vi "Test Async Handler Warning Logged.vi"(8 "error in (no error)":errorcluster, 11 "Test Case In":refnum<class "Async Handling Test.lvclass">) -> (0 "error out":errorcluster, 3 "Test Case Out":refnum<class "Async Handling Test.lvclass">)   [LabVIEW 2020, in "Async Handling Test.lvclass"]
uses:
  Async Handling Test.lvclass
  C:/Program Files (x86)/National Instruments/LabVIEW 2020/vi.lib/Astemes/LUnit/Test Case.lvclass
  Mock Async Handler Process/Mock Async Handler Process.lvclass
  C:/Git/astemes-triarc-framework/source/Framework/Process/Process.lvclass
  source/Framework Test Suite/Mock Log Handler/Mock Log Handler.lvclass
  C:/Git/astemes-triarc-framework/source/Framework/Logging/Logging.lvclass
  source/Framework/Process/Process.lvclass/Process.ctl
  <vilib>/Astemes/LUnit/Test Case.lvclass/Test Case.ctl
  01074fa8-ee8a-411d-bc8b-fc92c4f90959.vi
  source/Framework/Process/Public/Lifecycle/Get Lifecycle State.vi
  source/Framework/Process/Protected/Messaging/Send Message.vi
  source/Framework/Broadcast Event Helpers/Execution timer.vi
  source/Framework/Process/Private/SubVIs/Wait for finish.vi
  source/Framework/Process/Private/SubVIs/Set Lifecycle State.vi
  <vilib>/Astemes/LUnit/Palette/Pass.vi
  <vilib>/Astemes/LUnit/Palette/Fail.vi
  <vilib>/Astemes/LUnit/Compare Variants.vi
  <vilib>/Astemes/LUnit/Describe Comparison.vi
  <vilib>/Astemes/LUnit/Set Assertion Type.vi
  <vilib>/Utility/error.llb/Clear Errors.vi
  source/Framework/Process/Private/SubVIs/Handle Debug Data.vi
  <vilib>/Astemes/LUnit/Add test result.vi
  <vilib>/Astemes/LUnit/Variant to string.vi
  source/Framework/Logging/Log Debug.vi
  <vilib>/AdvancedString/1D String Array to Delimited String.vi
  <vilib>/Utility/High Resolution Relative Seconds.vi
  <vilib>/Astemes/LUnit/LUnit Record Assertion Result.vi
  <vilib>/Astemes/LUnit/LUnit Aggregate Assertion Results.vi
  <vilib>/Astemes/LUnit/Method Result/LUnit Merge Status.vi
  <vilib>/Astemes/LUnit/LUnit Concatenate result strings.vi
  <vilib>/Utility/error.llb/Error Cluster From Error Code.vi
  source/Framework/Process/Public/Read Name.vi
  source/Framework/Broadcast Event Helpers/Dequeue Broadcast Message.vi
  <vilib>/Utility/Data Type/Get Type Information.vi
  <vilib>/Utility/LVClass/Get LV Class Name.vi
  source/Framework/Process/Process.lvclass
  source/Framework/Broadcast Event Helpers/Broadcast Event Helpers.lvlib
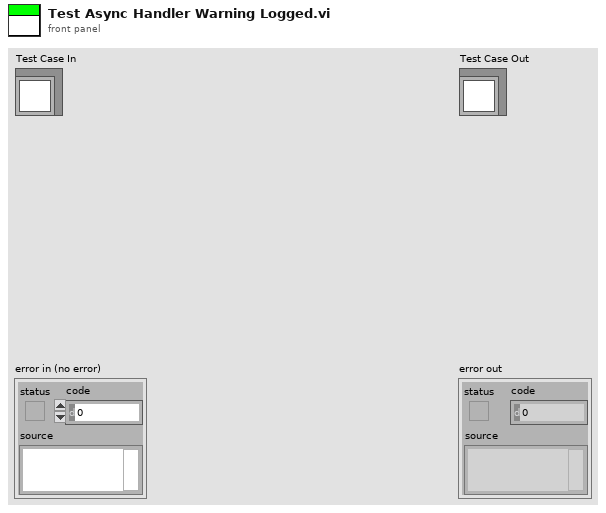
[diagram p1: front panel]
types:
  T1 = typedef "Mock Log Handler.lvclass/Log Entry.ctl" = cluster{"Level":string, "Source":string, "Message":string}
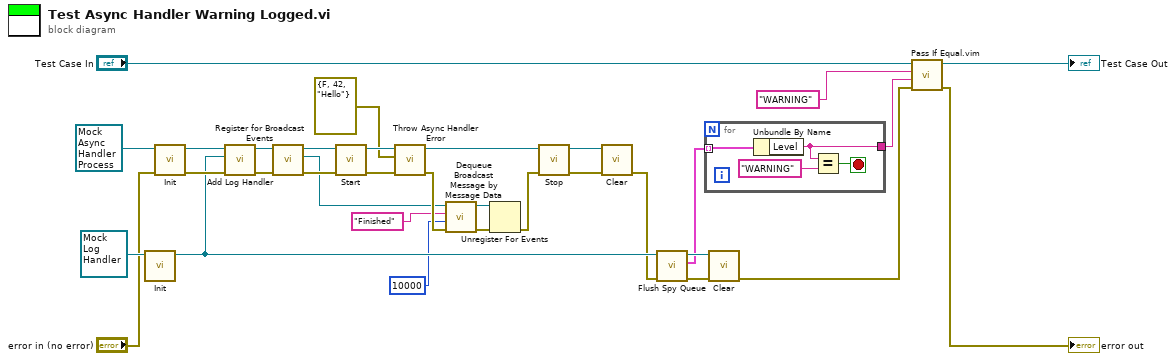
[diagram p0: block diagram]
diagram:
  n1 = call-dynamic "Init.vi"("Mock Log Handler In"=refnum<class "Mock Log Handler.lvclass"> refnum ("Mock Log Handler.lvclass")) -> ("Mock Log Handler Out"=w20:refnum<class "Mock Log Handler.lvclass">)  [unwired: 9 in, 1 out]
  n2 = call-dynamic "Init.vi"("error in (no error)"="error in (no error)", "Process In"=refnum<class "Mock Async Handler Process.lvclass"> refnum ("Mock Async Handler Process.lvclass")) -> ("error out"=w30:errorcluster, "Process Out"=w25:refnum<class "Mock Async Handler Process.lvclass">)  [unwired: 8 in]
  n3 = call "Add Log Handler.vi"("error in (no error)"=w30, "Log Handler"=w20, "Process In"=w25) -> ("error out"=w26:errorcluster, "Process Out"=w9:refnum<class "Mock Async Handler Process.lvclass">)  [unwired: 7 in]
  n4 = call "Register for Broadcast Events.vi"("error in (no error)"=w26, "Process In"=w9) -> ("error out"=w10:errorcluster, "Event Registration Refnum Out"=w5:refnum<event-registration>, "Process Out"=w8:refnum<class "Mock Async Handler Process.lvclass">)  [unwired: 7 in]
  n5 = call "Start.vi"("error in (no error)"=w10, "Process In"=w8) -> ("error out"=w29:errorcluster, "Process Out"=w22:refnum<class "Mock Async Handler Process.lvclass">)  [unwired: 7 in, 1 out]
  n6 = call "Throw Async Handler Error.vi"("error in (no error)"=w29, "Error"=errorcluster {"status"=FALSE, "code"=42, "source"="Hello"}, "Mock Async Handler Process in"=w22) -> ("error out"=w6:errorcluster, "Mock Async Handler Process out"=w24:refnum<class "Mock Async Handler Process.lvclass">)  [unwired: 7 in]
  n7 = call "Dequeue Broadcast Message by Message Data.vi"("error in (no error)"=w6, "Timeout (-1)"=10000, "Message Data"="Finished" ("Message"), "Event Registration Refnum"=w5) -> ("error out"=w7:errorcluster, "Event Registration Refnum Out"=w1:refnum<event-registration>)  [unwired: 3 in, 3 out]
  n8 = Unregister For Events(event registration refnum=w1, error in=w7) -> (error out=w2:errorcluster)
  n9 = call "Stop.vi"("error in (no error)"=w2, "Process In"=w24) -> ("error out"=w27:errorcluster, "Process Out"=w28:refnum<class "Mock Async Handler Process.lvclass">)  [unwired: 7 in, 1 out]
  n10 = call-dynamic "Clear.vi"("error in (no error)"=w27, "Process In"=w28) -> ("error out"=w18:errorcluster)  [unwired: 9 in]
  n11 = call "Flush Spy Queue.vi"("error in (no error)"=w18, "Mock Log Handler in"=w20) -> ("error out"=w17:errorcluster, "remaining elements"=w16:T1[], "Mock Log Handler out"=w19:refnum<class "Mock Log Handler.lvclass">)  [unwired: 7 in]
  n12 = for {
    tunnel: w16 -> [w37] mode=indexing
    tunnel: [w34] -> w14
    stop <- w35 stop-if-true
    n13 = Unbundle By Name(w37) -> ("Level"=w34:string)
    n14 = Equal?(x=w34, y="WARNING") -> (x = y?=w35:bool)
  }
  n15 = call-dynamic "Clear.vi"("error in (no error)"=w17, "Mock Log Handler In"=w19) -> ("error out"=w12:errorcluster)  [unwired: 9 in]
  n16 = call "Pass If Equal.vim"("error in (no error)"=w12, "Actual"=w14, "Expected"="WARNING" ("y"), "LUnit Test Case In"="Test Case In") -> ("error out"=→"error out":errorcluster, "LUnit Test Case Out"=→"Test Case Out":refnum<class "Async Handling Test.lvclass">)  [unwired: 6 in]
